vi "Update SSM.vi"(8 "error in":errorcluster, 10 "SSM value":u8 format="%02b", 11 "32-bit Word in":refnum<class "32-bit Word.lvclass">) -> (0 "error out":errorcluster, 3 "32-bit Word out":refnum<class "32-bit Word.lvclass">)   [LabVIEW 2020, in "32-bit Word.lvclass"]
uses:
  32-bit Word.lvclass
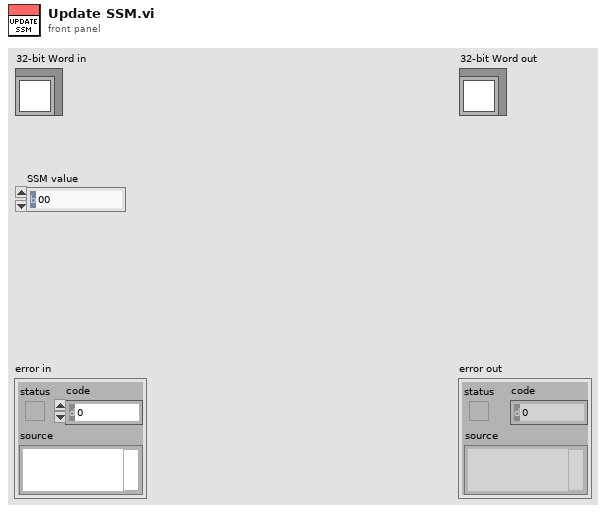
[diagram p1: front panel]
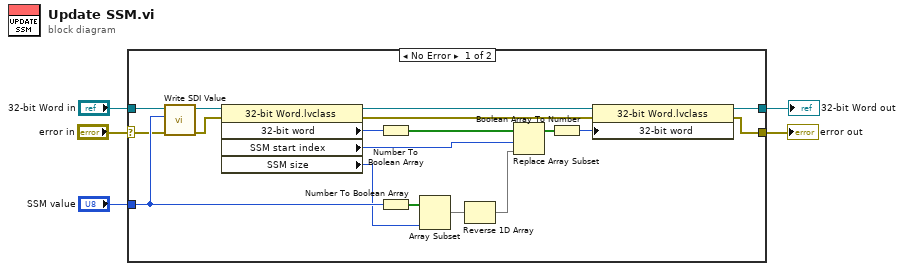
[diagram p0: block diagram]
diagram:
  n1 = case shown="No Error" "error in" {
    selector: "error in" -> [w8 w25]
    tunnel: [w7 w25] -> w4
    tunnel: [w9 w24] -> w2
    tunnel: "32-bit Word in" -> [w23 w24]
    tunnel: "SSM value" -> [w20 _]
    frame No Error {
      n2 = call "Write SDI Value.vi"("error in"=w8, "SDI value"=w20, "32-bit Word in"=w23) -> ("error out"=w21:errorcluster, "32-bit Word out"=w22:refnum<class "32-bit Word.lvclass">)  [unwired: 7 in]
      n3 = property class="32-bit Word.lvclass"(reference=w22, error in=w21) -> (reference out=w12:refnum<class "32-bit Word.lvclass">, error out=w13:errorcluster, "32-bit word"=w17:u32, "SSM start index"=w15:i32, "SSM size"=w19:i32)
      n4 = Number To Boolean Array(number=w17) -> (Boolean array=w16:bool[])
      n5 = Number To Boolean Array(number=w20) -> (Boolean array=w18:bool[])
      n6 = Array Subset(array=w18, length=w19) -> (w14:bool[])  [unwired: 1 in]
      n7 = Reverse 1D Array(array=w14) -> (reversed array=w6:bool[])
      n8 = Replace Array Subset(array=w16, new element=w6, index=w15) -> (w11:bool[])
      n9 = Boolean Array To Number(Boolean array=w11) -> (number=w10:u32)
      n10 = property class="32-bit Word.lvclass"(reference=w12, error in=w13, "32-bit word"=w10) -> (reference out=w9:refnum<class "32-bit Word.lvclass">, error out=w7:errorcluster)
    }
    frame Error {
    }
  }
  "error out" <- w4
  "32-bit Word out" <- w2
